vi "DCTSrXTemplate.vi"(3 ";error in (no error)":errorcluster, 5 ";Type":i32, 6 ";DataIn":string) -> (0 "Error (out)":errorcluster, 1 "Time Stamp":timestamp, 2 ";Data out":string)   [LabVIEW 2017]
uses:
  <vilib>/variable/detnetvar/DSV init parameters.ctl
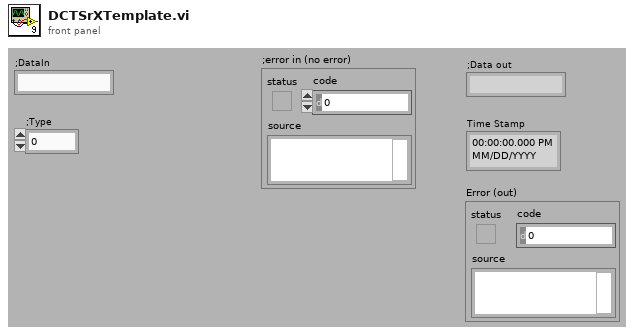
[diagram p1: front panel]
types:
  T1 = typedef "DSV init parameters.ctl" = cluster{"refIndex in":i32, "MAC Address":string, "NodeId":string, "SMB block Offset (us)":i32, "Max Variable Length":i32, "Sub Items":i32, "Item Size (bytes)":u16, "Index":i32, "SMB item Data Offset (bytes)":i32, "Timing Source Name":string, "Node is owner?":bool, "Num Items":i32, "Start Slot (us) ":i32, "GUID":string, "Reserved":string, "Cycle time (us)":i32, "Master?":bool, "Max Overall\n Message Length ":i32, "Version Count":u32, "SMB Start Times (other nodes)":i32[], "Network Speed":enum16{"100 MBit", "1 GBit"}, "SMB Variable":bool}
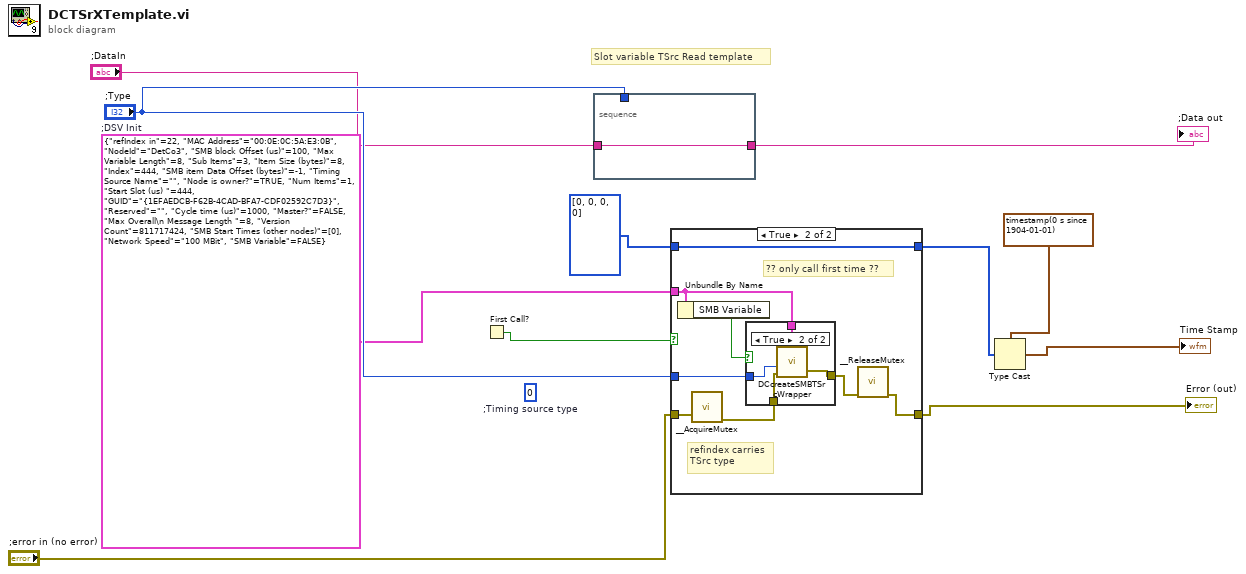
[diagram p0: block diagram]
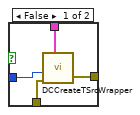
[diagram p3: hidden frame]
diagram:
  w1 = T1 {"refIndex in"=22, "MAC Address"="00:0E:0C:5A:E3:0B", "NodeId"="DetCo3", "SMB block Offset (us)"=100, "Max Variable Length"=8, "Sub Items"=3, "Item Size (bytes)"=8, "Index"=444, "SMB item Data Offset (bytes)"=-1, "Timing Source Name"="", "Node is owner?"=TRUE, "Num Items"=1, "Start Slot (us) "=444, "GUID"="{1EFAEDCB-F62B-4CAD-BFA7-CDF02592C7D3}", "Reserved"="", "Cycle time (us)"=1000, "Master?"=FALSE, "Max Overall\n Message Length "=8, "Version Count"=811717424, "SMB Start Times (other nodes)"=[0], "Network Speed"=enum."100 MBit", "SMB Variable"=FALSE}  # ;DSV Init
  (unwired) 0  # ;Timing source type
  # "Slot variable TSrc Read template"
  n1 = First Call?() -> (First Call?: T/F=w2:bool)
  n2 = stacked-sequence {
    tunnel: ";DataIn" -> [w12]
    tunnel: [w12] -> w8
    tunnel: ";Type" -> [_]
    frame #0 {
    }
  }
  ";Data out" <- w8
  n3 = case shown="True" w2 {
    tunnel: ";error in (no error)" -> [w14 w22]
    tunnel: [w14 w19] -> w3
    tunnel: w1 -> [_ w16]
    tunnel: [w13 w18] -> w9
    tunnel: u32[] [0, 0, 0, 0] ("Timestamp") -> [w13 w18]
    tunnel: ";Type" -> [_ w17]
    frame False {
    }
    frame True {
      # "?? only call first time ??"
      # "refindex carries\nTSrc type"
      n4 = Unbundle By Name(w16) -> ("SMB Variable"=w15:bool)
      n5 = call <vilib>:"__AcquireMutex.vi"("Error"=w22) -> ("Error (out)"=w21:errorcluster)  [unwired: 10 in]
      n6 = case shown="True" w15 {
        tunnel: w16 -> [w26 w30]
        tunnel: w21 -> [w25 w29]
        tunnel: [w24 w28] -> w20
        tunnel: w17 -> [w23 w27]
        frame False {
          n7 = call <vilib>:"DCCreateTSrcWrapper.vi"(";Init"=w26, ";error in (no error)"=w25, ";Timing source type"=w23) -> ("error out"=w24:errorcluster)  [unwired: 3 in, 1 out]
        }
        frame True {
          n8 = call <vilib>:"DCcreateSMBTSrcWrapper.vi"(";Init"=w30, ";error in (no error)"=w29, ";Timing source type"=w27) -> ("error out"=w28:errorcluster)  [unwired: 3 in, 1 out]
        }
      }
      n9 = call <vilib>:"__ReleaseMutex.vi"("Error"=w20) -> ("Error (out)"=w19:errorcluster)  [unwired: 10 in]
    }
  }
  "Error (out)" <- w3
  n10 = Type Cast(type=timestamp(0 s since 1904-01-01), x=w9) -> (*(type *) &x=→"Time Stamp":timestamp)
